vi "EJEM15.vi"() -> ()   [LabVIEW 2013]
panel:
  out "element":dbl
  in  "array":dbl[](array[numeric])
  out "size(s)":i32
  out "index of element":i32
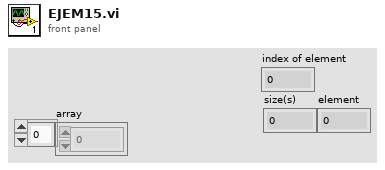
[diagram p1: front panel]
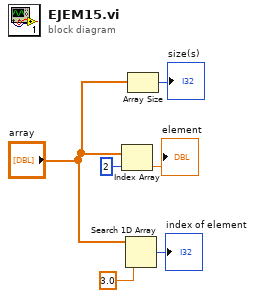
[diagram p0: block diagram]
diagram:
  n1 = Index Array(array="array", index=2) -> (element=→"element":dbl)
  n2 = Search 1D Array(1D array="array", element=3.0) -> (index of element=→"index of element":i32)  [unwired: 1 in]
  n3 = Array Size(array="array") -> (size(s)=→"size(s)":i32)
